vi "AlazarSetCaptureClock.vi"(0 "Handle":u64, 1 "Source":u32(ring)=1 items=["Internal"=1, "Fast External"=2, "Medium External"=3, "Slow External"=4, "External AC"=5, "External DC"=6, "External 10MHz"=7], 2 "Sample Rate":u32(ring)=30 items=["1 kS/s"=1, "2 kS/s"=2, "5 kS/s"=4, "10 kS/s"=8, "20 kS/s"=10, "50 kS/s"=12, "100 kS/s"=14, "200 kS/s"=16, "500 kS/s"=18, "1 MS/s"=20, "2 MS/s"=24, "5 MS/s"=26, "10 MS/s"=28, "20 MS/s"=30, "25 MS/s"=33, "50 MS/s"=34, "100 MS/s"=36, "125 MS/s"=37, "160 MS/s"=38, "180 MS/s"=39, "250 MS/s"=43, "500 MS/s"=48, "800 MS/s"=50, "1000 MS/s"=53, "1200 MS/s"=55, "1500 MS/s"=58, "1800 MS/s"=61], 3 "Edge":u32(ring) items=["Rising", "Falling"], 4 "Decimation":u32, 5 "error in (no error)":errorcluster) -> (14 "Handle":u64, 18 "Return Code":u32, 19 "error out":errorcluster)   [LabVIEW 2023]
doc: "Configure sample clock source, edge, and decimation."
uses:
  ATSApi.dll
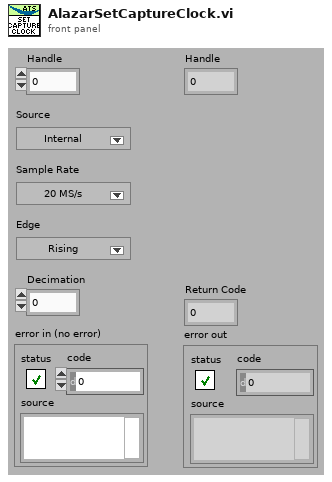
[diagram p1: front panel]
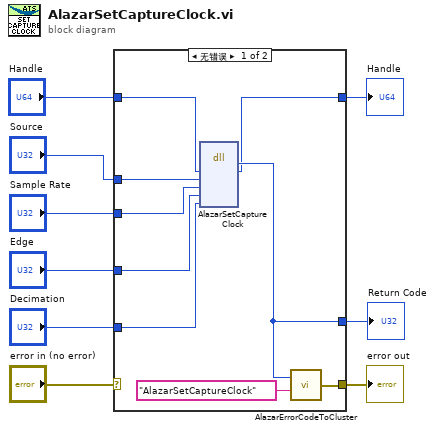
[diagram p0: block diagram]
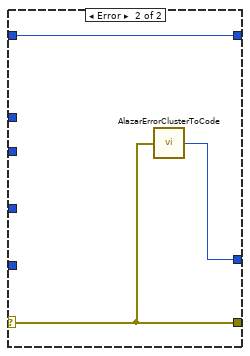
[diagram p2: hidden frame]
diagram:
  n1 = case shown="无错误" "error in (no error)" {
    selector: "error in (no error)" -> [_ w21]
    tunnel: [w15 w21] -> w8
    tunnel: [w17 w20] -> w7
    tunnel: "Handle" -> [w18 w19]
    tunnel: [w14 w19] -> w5
    tunnel: "Source" -> [w13 _]
    tunnel: "Sample Rate" -> [w12 _]
    tunnel: "Edge" -> [w11 _]
    tunnel: "Decimation" -> [w10 _]
    frame No Error {
      n2 = dll-call lib="ATSApi.dll" fn="AlazarSetCaptureClock"("handle"=w18, "source"=w13, "sampleRate"=w12, "edge"=w11, "decimation"=w10) -> ("return type"=w17:u32, "handle"=w14:u64)  [unwired: 7 in, 2 out]
      n3 = call "AlazarErrorCodeToCluster.vi"("Message"="AlazarSetCaptureClock", "Error Code"=w17) -> ("error out"=w15:errorcluster)
    }
    frame Error {
      n4 = call "AlazarErrorClusterToCode.vi"("error in (no error)"=w21) -> ("Error Code"=w20:u32)
    }
  }
  "Handle" <- w5
  "error out" <- w8
  "Return Code" <- w7
